vi "Add Remove Test.vi"() -> (0 "error out":errorcluster, 1 "Pass":bool, 2 "Success Delete":bool, 3 "Success ADD":bool)   [LabVIEW 2021, in "Multiplexer tests.lvlib"]
doc: "Tests the Add Line and Remove Line functions."
uses:
  Multiplexer tests.lvlib
  <vilib>/NI/Tag Bus/tag/Data Type.ctl
  configuration/Line.ctl
  <vilib>/NI/Tag Bus Module Framework/channel/TBM channel.lvclass
  configuration/permissions.ctl
  configuration/Multiplexer configuration.lvclass
  <vilib>/NI/Tag Bus/tag/tag descriptor.lvclass
panel:
  out "Deleted Line":string
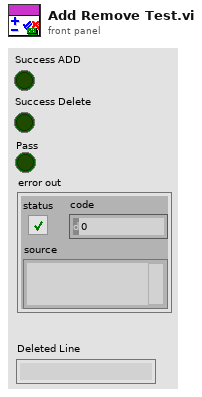
[diagram p1: front panel]
types:
  T1 = typedef "Multiplexer configuration.lvclass/permissions.ctl" = enum32{"Read from HW", "Write to HW"}
  T2 = typedef "Multiplexer configuration.lvclass/Line.ctl" = cluster{"A":refnum<class "TBM channel.lvclass">, "B":refnum<class "TBM channel.lvclass">, "Select":refnum<class "TBM channel.lvclass">, "Output":refnum<class "TBM channel.lvclass">}
  T3 = typedef "tag bus.lvlib/tag descriptor.lvclass/Data Type.ctl" = enum16{"Double", "Single", "I64", "I32", "I16", "I8", "U64", "U32", "U16", "U8", "Boolean", "String", "Array of Double", "Array of Single", "Array of I64", "Array of I32", "Array of I16", "Array of I8", "Array of U64", "Array of U32", "Array of U16", "Array of U8", "Array of Boolean", "Array of String"}
  T4 = typedef "TBM channel.lvclass/channel classification.ctl" = enum16{"input data", "output data", "processing parameter", "processing result"}
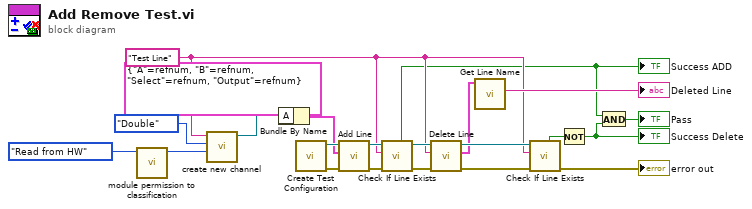
[diagram p0: block diagram]
diagram:
  w4 = "Test Line" ("channel name")
  n1 = call "module permission to classification.vi"("display permissions"=permissions."Read from HW") -> ("channel classification"=w20:T4)  [unwired: 10 in]
  n2 = call <vilib>:"create new channel.vi"("channel classification"=w20, "data type"=Data_Type."Double", "channel name"=w4) -> ("channel"=w21:refnum<class "TBM channel.lvclass">)  [unwired: 8 in]
  n3 = Bundle By Name(cluster=T2 {"A"=refnum, "B"=refnum, "Select"=refnum, "Output"=refnum} ("Line"), "A"=w21) -> (w18:T2)
  n4 = call "Create Test Configuration.vi"() -> ("error out"=w12:errorcluster, "Module Configuration"=w22:refnum<class "Multiplexer configuration.lvclass">)  [unwired: 6 in, 4 out]
  n5 = call "Add Line.vi"("error in"=w12, "Line"=w18, "Multiplexer configuration in"=w22) -> ("error out"=w14:errorcluster, "Multiplexer configuration out"=w16:refnum<class "Multiplexer configuration.lvclass">)  [unwired: 6 in, 1 out]
  n6 = call-dynamic "Check If Line Exists.vi"("error in"=w14, "Name to Locate"=w4, "Multiplexer configuration in"=w16) -> ("error out"=w13:errorcluster, "Multiplexer configuration out"=w15:refnum<class "Multiplexer configuration.lvclass">, "Found?"=w1:bool)  [unwired: 4 in, 2 out]
  "Success ADD" <- w1
  n7 = call "Delete Line.vi"("error in"=w13, "Line Name"=w4, "Multiplexer configuration in"=w15) -> ("error out"=w11:errorcluster, "Deleted Line"=w6:T2, "Multiplexer configuration out"=w9:refnum<class "Multiplexer configuration.lvclass">)  [unwired: 6 in]
  n8 = call "Get Line Name.vi"("Line in"=w6) -> ("Name"=→"Deleted Line":string)  [unwired: 8 in, 2 out]
  n9 = call-dynamic "Check If Line Exists.vi"("error in"=w11, "Name to Locate"=w4, "Multiplexer configuration in"=w9) -> ("error out"=→"error out":errorcluster, "Found?"=w8:bool)  [unwired: 4 in, 3 out]
  n10 = Not(x=w8) -> (.not. x?=w2:bool)
  "Success Delete" <- w2
  n11 = And(x=w1, y=w2) -> (x .and. y?=→"Pass":bool)
